vi "Get-all-param-groups-names.vi"() -> (3 "Param groups":T1[](array[typedef]))   [LabVIEW 2013, in "CameraVision.lvlib" / "CV-UI.lvclass"]
uses:
  CV-UI.lvclass
  Parameter-group-names.ctl
panel:
  in  "Praram group refs":T1
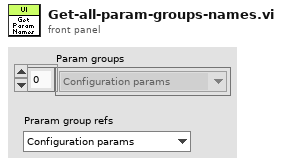
[diagram p1: front panel]
types:
  T1 = typedef "CameraVision.lvlib/CV-UI.lvclass/Parameter-group-names.ctl" = enum16{"Configuration params", "Acquisition params", "Correction params", "Analysis params", "Temperature params", "Mapping params", "Storage params", "Filter params"}
  T2 = typedef "CameraVision.lvlib/CV-UI.lvclass/Parameter-refs.ctl" = enum16{"Configuration params", "Acquisition params", "Correction params", "Analysis params", "Temperature params", "Mapping params", "Storage params", "Filter params"}
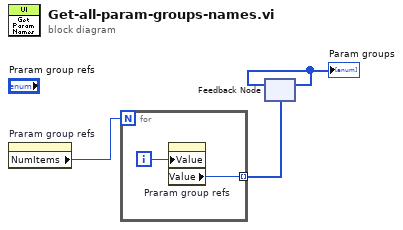
[diagram p0: block diagram]
diagram:
  n1 = property on="Praram group refs" class="Enum (strict)"() -> ("NumItems"=w2:u32)  [unwired: 2 in, 2 out]
  n2 = for {
    N: w2 -> [_]
    tunnel: [w4] -> w1 mode=indexing
    i -> [w5]
    n3 = property on="Praram group refs" class="Enum (strict)"("Value"=w5) -> ("Value"=w4:T2)  [unwired: 2 in, 2 out]
  }
  n4 = feedback #1(w1) -> (w3:T2[])
  "Param groups" <- w3
  n5 = feedback-in #1(w3) -> ()
